vi "Transmit Messages with Rate-based Schedule2.vi"() -> ()   [LabVIEW 2023]
doc: "This program opens the specified card, builds a transmit schedule \nusing transmit interval information in the channel configuration file,\nand then transmits the messages with changing data."
uses:
  <instrlib>/BTICardLib/Private/Initialize By Card Number and Core Number.vi
  <instrlib>/BTICardLib/Private/Configure Core From XML.vi
  <instrlib>/BTI429Lib/Private/Tx/Configure/Configure Tx Channel From XML.vi
  <instrlib>/BTI429Lib/Private/Core/Action-Status/Start All Tx Channels.vi
  <instrlib>/BTI429Lib/Private/Core/Action-Status/Stop All Tx Channels.vi
  <instrlib>/BTICardLib/BTICardLV.lvlib
  <instrlib>/BTI429Lib/BTI429LV.lvlib
panel:
  in  "Tab Control":enum32{"Egi1", "Egi2", "Esis"}(tab)
  out "Egi1 Pitch Angle Value OLD":u32 format="%.0b"
  in  "Egi1 Pitch Angle":dbl
  in  "Egi1 Roll Angle":dbl
  out "Egi1 Roll Angle Value OLD":u32 format="%.0b"
  out "Egi1 Roll Angle Value NEW":u32 format="%08x"
  out "Egi1 Pitch Angle Value NEW":u32 format="%08x"
  out "Egi1 Pitch Rate Value OLD":u32 format="%.0b"
  in  "Egi1 Pitch Rate":dbl
  in  "Egi1 Roll Rate":dbl
  out "Egi1 Roll Rate Value OLD":u32 format="%.0b"
  out "Egi1 Roll Rate Value NEW":u32 format="%08x"
  out "Egi1 Pitch Rate Value NEW":u32 format="%08x"
  in  "Egi1 Yaw Rate":dbl
  out "Egi1 Yaw Rate Value OLD":u32 format="%08b"
  out "Egi1 Yaw Rate Value NEW":u32 format="%08x"
  out "Egi1 Pitch Angle Range Message":string
  out "Egi1 Roll Angle Range Message":string
  out "Egi1 Roll Rate Range Message":string
  out "Egi1 Yaw Rate Range Message":string
  out "Egi1 Pitch Rate Range Message":string
  in  "Egi1 Pitch Angle Valid":u16
  in  "Egi1 Pitch Rate Valid":u16
  in  "Egi1 Roll Rate Valid":u16
  in  "Egi1 Yaw Rate Valid":u16
  in  "Egi1 Roll Angle Valid":u16
  in  "Egi2 Pitch Angle":dbl
  in  "Egi2 Roll Angle":dbl
  in  "Egi2 Roll Angle Valid":u16
  in  "Egi2 Pitch Angle Valid":u16
  out "Egi2 Pitch Angle Value OLD":u32 format="%.0b"
  out "Egi2 Roll Angle Value NEW":u32 format="%08b"
  out "Egi2 Pitch Angle Value NEW":u32 format="%08b"
  out "Egi2 Roll Angle Range Message":string
  out "Egi2 Pitch Angle Range Message":string
  out "Egi2 Roll Angle Value OLD":u32 format="%.0b"
  in  "Egi2 Yaw Rate Valid":u16
  in  "Egi2 Roll Rate Valid":u16
  in  "Egi2 Roll Rate":dbl
  in  "Egi2 Pitch Rate Valid":u16
  in  "Egi2 Yaw Rate":dbl
  in  "Egi2 Pitch Rate":dbl
  out "Egi2 Pitch Rate Value OLD":u32 format="%.0b"
  out "Egi2 Pitch Rate Range Message":string
  out "Egi2 Pitch Rate Value NEW":u32 format="%08b"
  out "Egi2 Roll Rate Range Message":string
  out "Egi2 Roll Rate Value OLD":u32 format="%.0b"
  out "Egi2 Roll Rate Value NEW":u32 format="%08b"
  out "Egi2 Yaw Rate Value OLD":u32 format="%08b"
  out "Egi2 Yaw Rate Value NEW":u32 format="%08b"
  out "Egi2 Yaw Rate Range Message":string
  in  "Esis Pitch Angle":dbl
  in  "Esis Roll Angle":dbl
  in  "Esis Pitch Rate":dbl
  in  "Esis Roll Rate":dbl
  in  "Esis Yaw Rate":dbl
  in  "Esis Pitch Angle Valid":u16
  in  "Esis Roll Angle Valid":u16
  in  "Esis Pitch Rate Valid":u16
  in  "Esis Roll Rate Valid":u16
  in  "Esis Yaw Rate Valid":u16
  out "Esis Yaw Rate Value NEW":u32 format="%08b"
  out "Esis Roll Rate Range Message":string
  out "Esis Yaw Rate Range Message":string
  out "Esis Pitch Angle Value NEW":u32 format="%08b"
  out "Esis Roll Angle Value NEW":u32 format="%08b"
  out "Esis Pitch Rate Value NEW":u32 format="%08b"
  out "Esis Roll Rate Value NEW":u32 format="%08b"
  out "Esis Pitch Angle Range Message":string
  out "Esis Roll Angle Range Message":string
  out "Esis Pitch Rate Range Message":string
  out "Esis Channel Xml Path":path
  in  "ESIS":string="ESIS Channel Config.xml"
  in  "Channel6":i32=22
  in  "EGI1":string="EGI1 Channel Config.xml"
  in  "EGI2":string="EGI2 Channel Config.xml"
  in  "CORE":string="Core Config.xml"
  in  "Channel0":i32=16
  in  "Channel3":i32=19
  out "Egi2 Channel Xml Path":path
  out "Core Xml Path":path
  out "Egi1 Channel Xml Path":path
  in  "Card number":i32
  in  "Core number":i32
  out "error out":errorcluster
  in  "stop":bool
  # "ARINC 429: Transmit Messages with Rate-based Schedule"
  # "©2016 Astronics Ballard Technology"
  # "This program opens the specified card, builds a transmit schedule \nusing transmit interval information in the channel configuration file,\nand then transmits the messages with changing data."
  # "Tx first channel Number is(P2Cable) ;\nChannel0 = 16;\nChannel1 = 17;\nChannel2 = 18;\nChannel3 = 19;\nChannel4 = 20;\nChannel5 = 21;\nChannel6 = 22;\nChannel7 = 23;\nChannel8 = 24;\nChannel9 = 25;\nChannel10 = 26;\nChannel11 = 27;\nChannel12 = 28;\nChannel13 = 29;\nChannel14 = 30;\nChannel15 = 31;\nChannel16 = 32;"
  # "Always Stop the card\nand Close the card when\ndone. Otherwise, the hardware\ncontinues to operate."
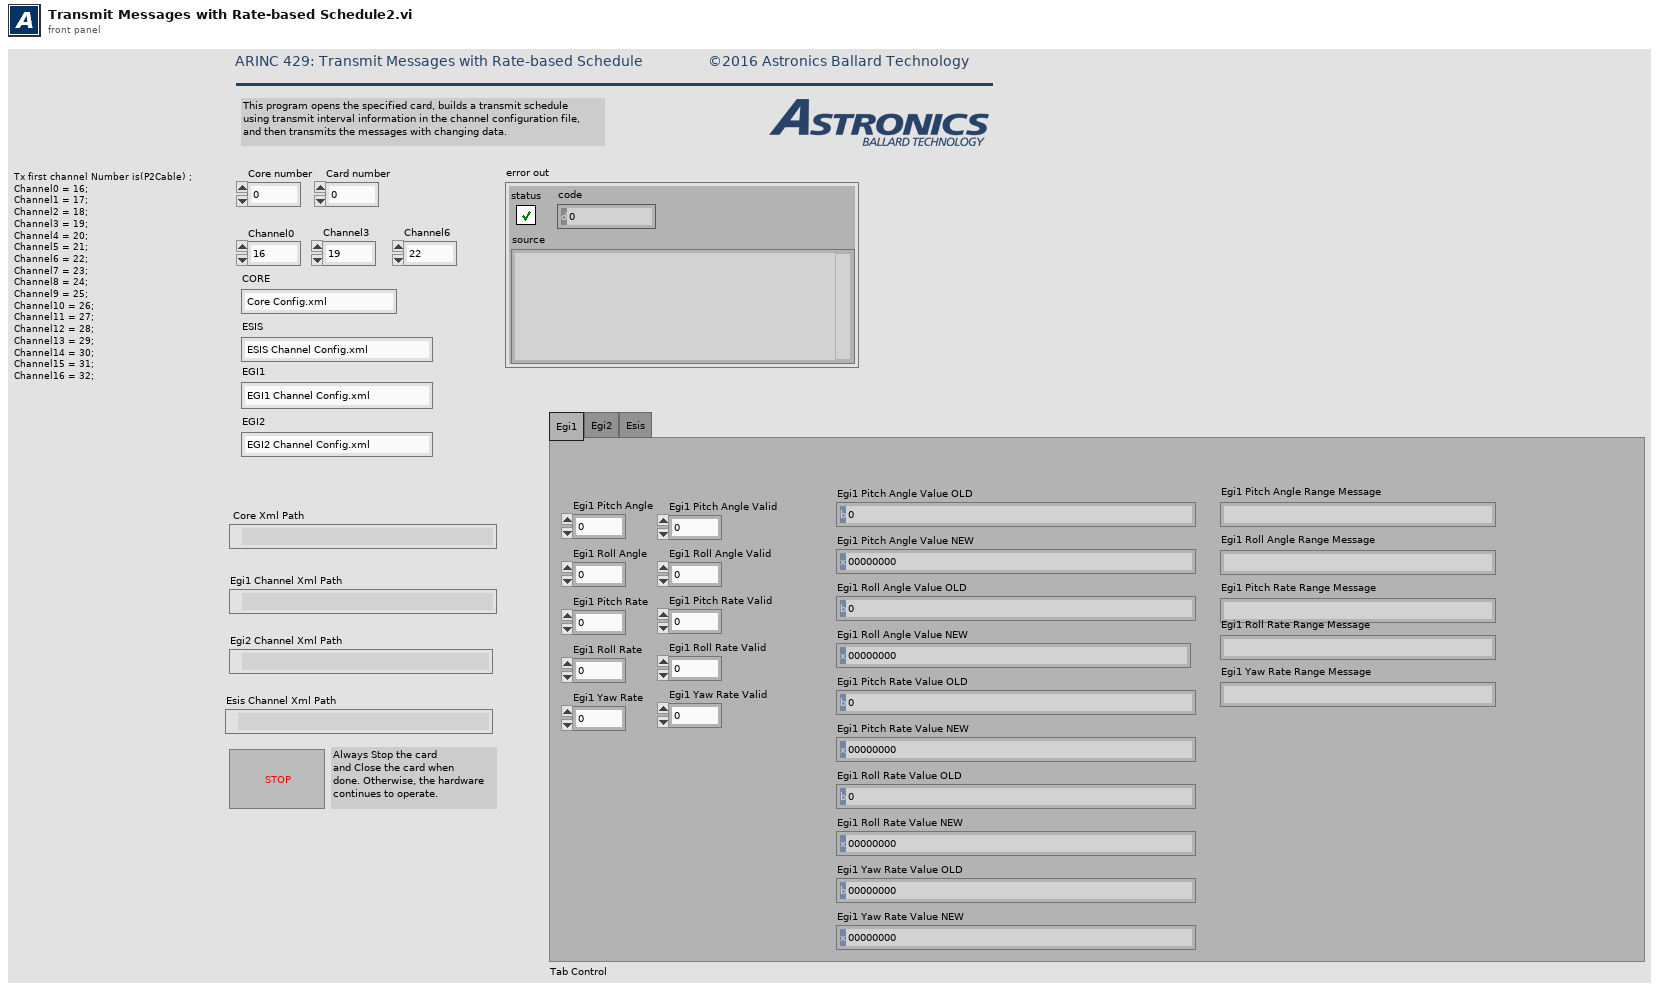
[diagram p1: front panel]
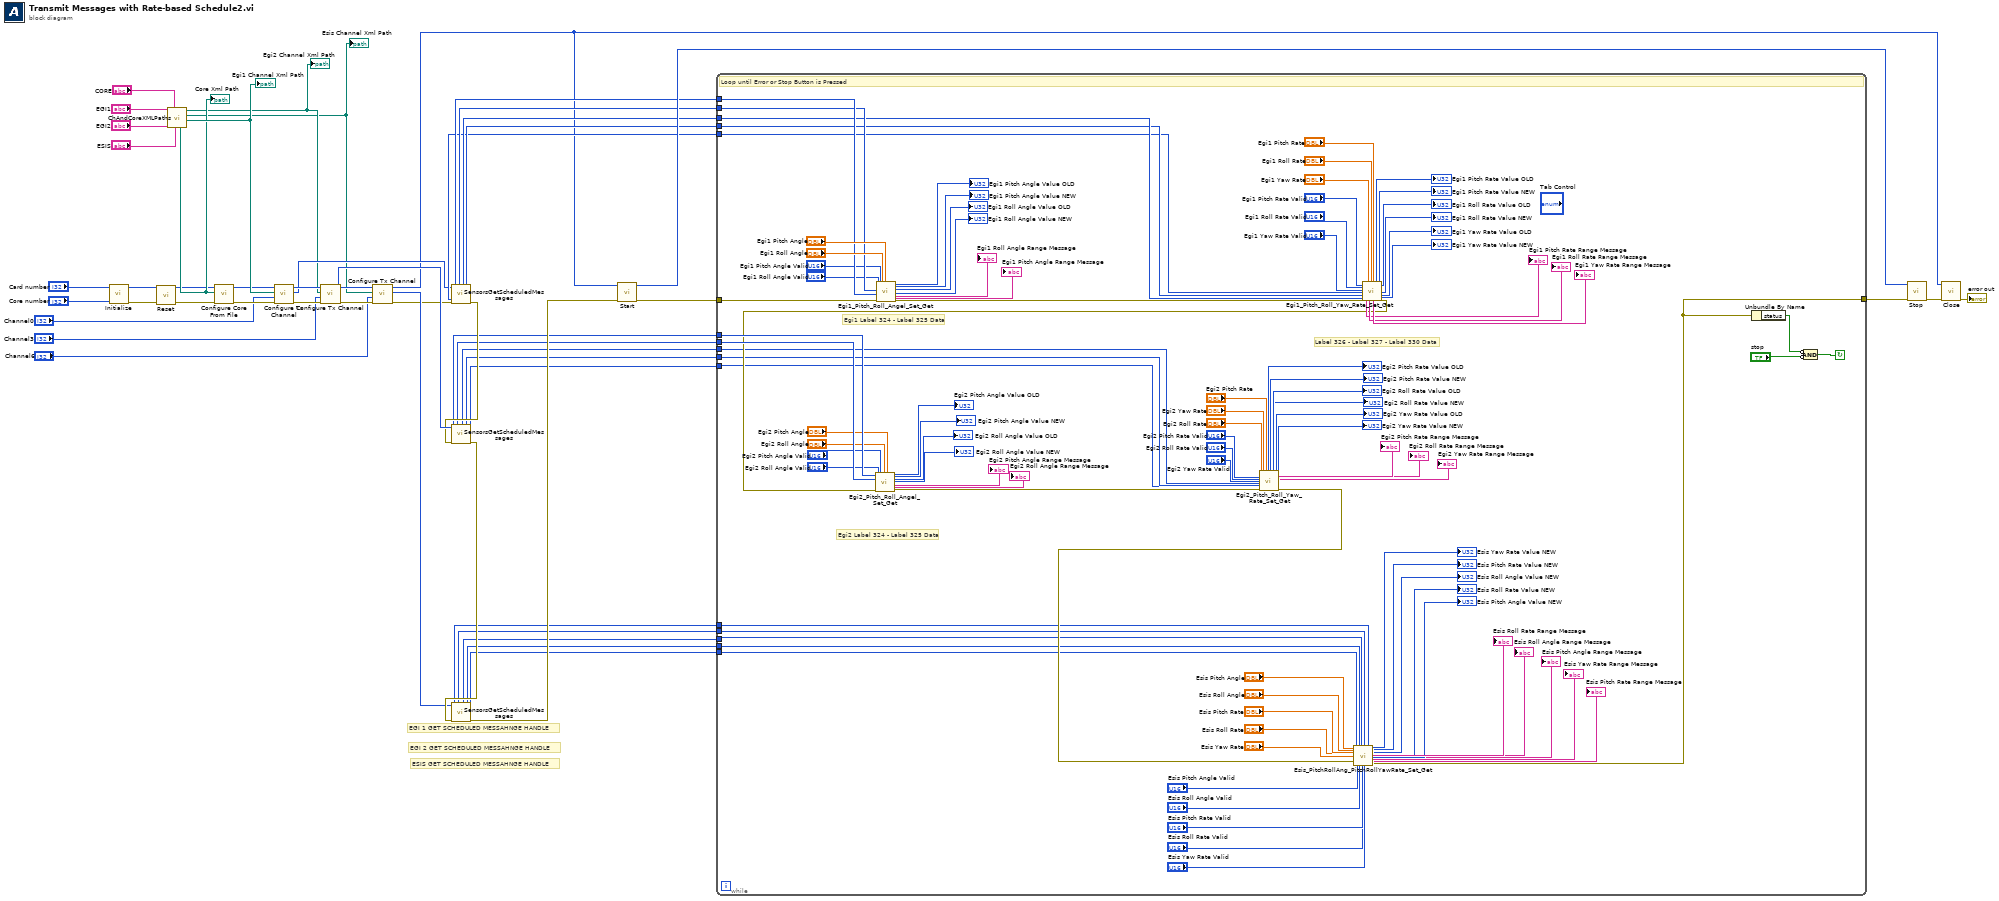
[diagram p0: block diagram]
diagram:
  # "ESIS GET SCHEDULED MESSAHNGE HANDLE"
  # "EGI 2 GET SCHEDULED MESSAHNGE HANDLE"
  # "EGI 1 GET SCHEDULED MESSAHNGE HANDLE"
  n1 = call-poly <instrlib>:"Initialize.vi"("core number"="Core number", "card number"="Card number") -> ("error out"=w39:errorcluster, "core handle out"=w40:u64)  [unwired: 8 in]
  n2 = call <instrlib>:"Reset.vi"("error in (no error)"=w39, "core handle in"=w40) -> ("error out"=w38:errorcluster, "core handle out"=w35:u64)  [unwired: 8 in]
  n3 = call "ChAndCoreXMLPaths.vi"("Esis"="ESIS", "Egi2"="EGI2", "Core"="CORE", "Egi1"="EGI1") -> ("Egi1 Xml Path"=w44:path, "Esis Xml Path"=w15:path, "Egi2 Xml Path"=w30:path, "Core Xml Path"=w43:path)  [unwired: 4 in]
  "Egi1 Channel Xml Path" <- w44
  "Core Xml Path" <- w43
  "Egi2 Channel Xml Path" <- w30
  "Esis Channel Xml Path" <- w15
  n4 = call-poly <instrlib>:"Configure Core From File.vi"("error in (no error)"=w38, "configuration file path"=w43, "core handle in"=w35) -> ("error out"=w45:errorcluster, "core handle out"=w34:u64)  [unwired: 7 in]
  n5 = call-poly <instrlib>:"Configure Tx Channel.vi"("error in (no error)"=w45, "channel number in"="Channel0", "configuration file path"=w44, "core handle in"=w34) -> ("error out"=w32:errorcluster, "channel handle out"=w31:u64, "core handle out"=w33:u64)  [unwired: 5 in]
  n6 = call-poly <instrlib>:"Configure Tx Channel.vi"("error in (no error)"=w32, "channel number in"="Channel3", "configuration file path"=w30, "core handle in"=w33) -> ("error out"=w24:errorcluster, "channel handle out"=w25:u64, "core handle out"=w23:u64)  [unwired: 5 in]
  n7 = call-poly <instrlib>:"Configure Tx Channel.vi"("error in (no error)"=w24, "channel number in"="Channel6", "configuration file path"=w15, "core handle in"=w23) -> ("error out"=w13:errorcluster, "channel handle out"=w16:u64, "core handle out"=w12:u64)  [unwired: 5 in]
  n8 = call "SensorsGetScheduledMessages.vi"("error in (no error)"=w13, "channel handle in"=w31) -> ("error out"=w19:errorcluster, "message handle out 4"=w37:u64, "message handle out 3"=w46:u64, "message handle out 5"=w36:u64, "message handle out 2"=w47:u64, "message handle out 1"=w48:u64)  [unwired: 3 in, 1 out]
  n9 = call "SensorsGetScheduledMessages.vi"("error in (no error)"=w19, "channel handle in"=w25) -> ("error out"=w18:errorcluster, "message handle out 4"=w8:u64, "message handle out 3"=w9:u64, "message handle out 5"=w7:u64, "message handle out 2"=w10:u64, "message handle out 1"=w11:u64)  [unwired: 3 in, 1 out]
  n10 = call "SensorsGetScheduledMessages.vi"("error in (no error)"=w18, "channel handle in"=w16) -> ("error out"=w17:errorcluster, "message handle out 4"=w3:u64, "message handle out 3"=w4:u64, "message handle out 5"=w2:u64, "message handle out 2"=w5:u64, "message handle out 1"=w6:u64)  [unwired: 3 in, 1 out]
  n11 = call-poly <instrlib>:"Start.vi"("error in (no error)"=w17, "core handle in"=w12) -> ("error out"=w51:errorcluster, "core handle out"=w49:u64)  [unwired: 8 in]
  n12 = while {
    tunnel: w51 -> [w141]
    tunnel: w48 -> [w134]
    tunnel: w47 -> [w133]
    tunnel: w46 -> [w119]
    tunnel: w37 -> [w118]
    tunnel: w36 -> [w117]
    tunnel: w11 -> [w112]
    tunnel: w10 -> [w111]
    tunnel: w9 -> [w84]
    tunnel: w8 -> [w83]
    tunnel: w7 -> [w82]
    tunnel: w6 -> [w57]
    tunnel: w5 -> [w56]
    tunnel: w4 -> [w55]
    tunnel: w3 -> [w54]
    tunnel: w2 -> [w53]
    tunnel: [w59] -> w1
    stop <- w144 continue-if-true
    # "Egi2 Label 324 - Label 325 Data"
    # "Label 326 - Label 327 - Label 330 Data"
    # "Egi1 Label 324 - Label 325 Data"
    # "Loop until Error or Stop Button is Pressed"
    n13 = call "Egi1_Pitch_Roll_Angel_Set_Get.vi"("Egi1 Roll Angle"="Egi1 Roll Angle", "Egi1 Roll Angle Valid"="Egi1 Roll Angle Valid", "message handle in 2"=w133, "message handle in1"=w134, "error in (no error)"=w141, "Egi1 Pitch Angle Valid"="Egi1 Pitch Angle Valid", "Egi1 Pitch Angle"="Egi1 Pitch Angle") -> ("Egi1 Roll Angle Range Message"=→"Egi1 Roll Angle Range Message":string, "Egi1 Pitch Angle Range Message"=→"Egi1 Pitch Angle Range Message":string, "Egi1 Roll Angle Value NEW"=→"Egi1 Roll Angle Value NEW":u32, "Egi1 Pitch Angle Value OLD"=→"Egi1 Pitch Angle Value OLD":u32, "Egi1 Pitch Angle Value NEW"=→"Egi1 Pitch Angle Value NEW":u32, "Egi1 Roll Angle Value OLD"=→"Egi1 Roll Angle Value OLD":u32, "error out"=w120:errorcluster)  [unwired: 6 in]
    n14 = call "Egi1_Pitch_Roll_Yaw_Rate_Set_Get.vi"("message handle in 3"=w117, "message handle in 2"=w118, "Egi1 Pitch Rate Valid"="Egi1 Pitch Rate Valid", "Egi1 Roll Rate Valid"="Egi1 Roll Rate Valid", "Egi1 Roll Rate"="Egi1 Roll Rate", "message handle in1"=w119, "Egi1 Yaw Rate Valid"="Egi1 Yaw Rate Valid", "error in (no error)"=w120, "Egi1 Yaw Rate"="Egi1 Yaw Rate", "Egi1 Pitch Rate"="Egi1 Pitch Rate") -> ("Egi1 Roll Rate Range Message"=→"Egi1 Roll Rate Range Message":string, "Egi1 Pitch Rate Range Message"=→"Egi1 Pitch Rate Range Message":string, "Egi1 Pitch Rate Value OLD"=→"Egi1 Pitch Rate Value OLD":u32, "Egi1 Yaw Rate Value NEW"=→"Egi1 Yaw Rate Value NEW":u32, "Egi1 Pitch Rate Value NEW"=→"Egi1 Pitch Rate Value NEW":u32, "Egi1 Roll Rate Value OLD"=→"Egi1 Roll Rate Value OLD":u32, "Egi1 Yaw Rate Range Message"=→"Egi1 Yaw Rate Range Message":string, "Egi1 Roll Rate Value NEW"=→"Egi1 Roll Rate Value NEW":u32, "Egi1 Yaw Rate Value OLD"=→"Egi1 Yaw Rate Value OLD":u32, "error out"=w108:errorcluster)  [unwired: 8 in]
    n15 = call "Egi2_Pitch_Roll_Angel_Set_Get.vi"("message handle in1"=w112, "Egi2 Pitch Angle Valid"="Egi2 Pitch Angle Valid", "message handle in 2"=w111, "Egi2 Pitch Angle"="Egi2 Pitch Angle", "Egi2 Roll Angle"="Egi2 Roll Angle", "error in (no error)"=w108, "Egi2 Roll Angle Valid"="Egi2 Roll Angle Valid") -> ("Egi2 Pitch Angle Value OLD"=→"Egi2 Pitch Angle Value OLD":u32, "Egi2 Roll Angle Value NEW"=→"Egi2 Roll Angle Value NEW":u32, "Egi2 Pitch Angle Value NEW"=→"Egi2 Pitch Angle Value NEW":u32, "Egi2 Roll Angle Range Message"=→"Egi2 Roll Angle Range Message":string, "Egi2 Pitch Angle Range Message"=→"Egi2 Pitch Angle Range Message":string, "Egi2 Roll Angle Value OLD"=→"Egi2 Roll Angle Value OLD":u32, "error out"=w81:errorcluster)  [unwired: 2 in]
    n16 = call "Egi2_Pitch_Roll_Yaw_Rate_Set_Get.vi"("Egi2 Yaw Rate Valid"="Egi2 Yaw Rate Valid", "Egi2 Roll Rate Valid"="Egi2 Roll Rate Valid", "message handle in 2"=w83, "Egi2 Roll Rate"="Egi2 Roll Rate", "Egi2 Pitch Rate Valid"="Egi2 Pitch Rate Valid", "error in (no error)"=w81, "message handle in 3"=w82, "message handle in1"=w84, "Egi2 Yaw Rate"="Egi2 Yaw Rate", "Egi2 Pitch Rate"="Egi2 Pitch Rate") -> ("Egi2 Pitch Rate Value OLD"=→"Egi2 Pitch Rate Value OLD":u32, "Egi2 Pitch Rate Range Message"=→"Egi2 Pitch Rate Range Message":string, "Egi2 Pitch Rate Value NEW"=→"Egi2 Pitch Rate Value NEW":u32, "Egi2 Roll Rate Range Message"=→"Egi2 Roll Rate Range Message":string, "Egi2 Roll Rate Value OLD"=→"Egi2 Roll Rate Value OLD":u32, "Egi2 Roll Rate Value NEW"=→"Egi2 Roll Rate Value NEW":u32, "Egi2 Yaw Rate Value OLD"=→"Egi2 Yaw Rate Value OLD":u32, "Egi2 Yaw Rate Value NEW"=→"Egi2 Yaw Rate Value NEW":u32, "Egi2 Yaw Rate Range Message"=→"Egi2 Yaw Rate Range Message":string, "error out"=w80:errorcluster)
    n17 = call "Esis_PitchRollAng_PitchRollYawRate_Set_Get.vi"("message handle in1"=w57, "message handle in 2"=w56, "message handle in 3"=w55, "message handle in 4"=w54, "message handle in 5"=w53, "Esis Pitch Angle"="Esis Pitch Angle", "Esis Roll Angle"="Esis Roll Angle", "Esis Pitch Rate"="Esis Pitch Rate", "Esis Roll Rate"="Esis Roll Rate", "Esis Yaw Rate"="Esis Yaw Rate", "Esis Pitch Angle Valid"="Esis Pitch Angle Valid", "Esis Roll Angle Valid"="Esis Roll Angle Valid", "Esis Pitch Rate Valid"="Esis Pitch Rate Valid", "Esis Roll Rate Valid"="Esis Roll Rate Valid", "Esis Yaw Rate Valid"="Esis Yaw Rate Valid", "error in (no error)"=w80) -> ("Esis Yaw Rate Value NEW"=→"Esis Yaw Rate Value NEW":u32, "Esis Roll Rate Range Message"=→"Esis Roll Rate Range Message":string, "Esis Yaw Rate Range Message"=→"Esis Yaw Rate Range Message":string, "Esis Pitch Angle Value NEW"=→"Esis Pitch Angle Value NEW":u32, "Esis Roll Angle Value NEW"=→"Esis Roll Angle Value NEW":u32, "Esis Pitch Rate Value NEW"=→"Esis Pitch Rate Value NEW":u32, "Esis Roll Rate Value NEW"=→"Esis Roll Rate Value NEW":u32, "Esis Pitch Angle Range Message"=→"Esis Pitch Angle Range Message":string, "Esis Roll Angle Range Message"=→"Esis Roll Angle Range Message":string, "Esis Pitch Rate Range Message"=→"Esis Pitch Rate Range Message":string, "error out"=w59:errorcluster)  [unwired: 1 in]
    n18 = Unbundle By Name(w59) -> ("status"=w58:bool)
    n19 = Compound Arithmetic op=AND(invert w58, invert "stop") -> (w144:bool)
  }
  n20 = call-poly <instrlib>:"Stop.vi"("error in (no error)"=w1, "core handle in"=w49) -> ("error out"=w20:errorcluster)  [unwired: 8 in, 1 out]
  n21 = call <instrlib>:"Close.vi"("error in (no error)"=w20, "core handle in"=w12) -> ("error out"=→"error out":errorcluster)  [unwired: 8 in, 1 out]
